vi "(SubVI) Test laser feedback performance .vi"(9 "Sampling rate (Hz)":dbl=20000.0, 10 "all rows":dbl[][](array[numeric]), 11 "Avg points":i32) -> (0 "Raw Data":dbl[](array[numeric]), 1 "Filtered QPD data":dbl[](array[numeric]), 2 "Time":dbl[](array[numeric]), 3 "Array":cluster{dbl[], "all rows":dbl[]}[](array[cluster]))   [LabVIEW 2014]
panel:
  in  "Filter type":T1(ring)
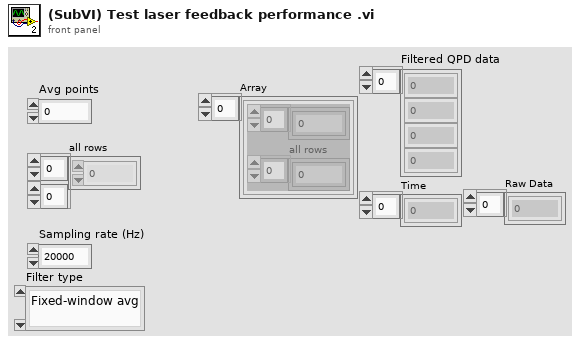
[diagram p1: front panel]
types:
  T1 = enum16{"Fixed-window avg", "Moving-window avg", "F+S-window avg", "S-G filter", "Fixed-window Median", "Moving-window Median "}
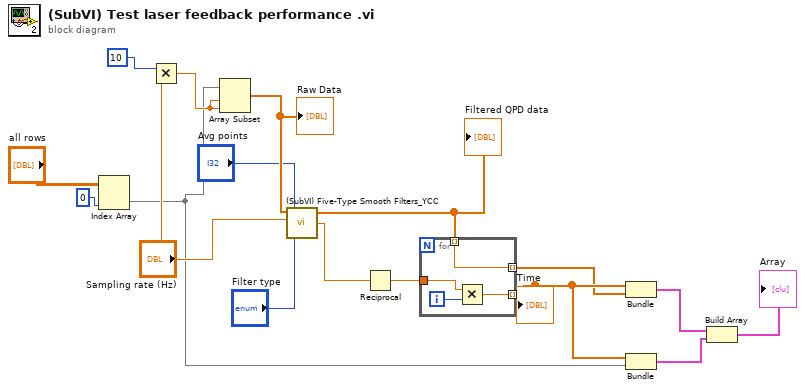
[diagram p0: block diagram]
diagram:
  n1 = Index Array(array="all rows", index (col)=0 ("index (row)")) -> (element=w13:dbl[])  [unwired: 1 in]
  n2 = Multiply(x=10 ("index"), y="Sampling rate (Hz)") -> (x*y=w16:dbl)
  n3 = Array Subset(array=w13, index=w16, length=w16) -> (w17:dbl[])
  "Raw Data" <- w17
  n4 = call "(SubVI) Five-Type Smooth Filters_YCC.vi"("Filter type"="Filter type", "Avg points"="Avg points", "Sampling rate (Hz)"="Sampling rate (Hz)", "QPD data"=w17) -> ("Sampling rate after filtering (Hz)"=w5:dbl, "Filtered QPD data"=w4:dbl[])  [unwired: 1 in]
  "Filtered QPD data" <- w4
  n5 = Reciprocal(x=w5) -> (1/x=w6:dbl)
  n6 = for {
    tunnel: [w21] -> w7 mode=indexing
    tunnel: w4 -> [w21] mode=indexing
    tunnel: w6 -> [w19]
    tunnel: [w18] -> w11 mode=indexing
    i -> [w20]
    n7 = Multiply(x=w19, y=w20) -> (x*y=w18:dbl)
  }
  "Time" <- w11
  n8 = Bundle(w11, w7) -> (w9:cluster{dbl[], dbl[]})  [unwired: 1 in]
  n9 = Bundle(w11, "all rows"=w13) -> (w10:cluster{dbl[], "all rows":dbl[]})  [unwired: 1 in]
  n10 = Build Array(w9, w10) -> (→"Array":cluster{dbl[], "all rows":dbl[]}[])
